vi "Get TimerDRV Period.vi"(11 "TimerDRV in":refnum<class "TimerDRV.lvclass">) -> (2 "TimerDRV Period":i64, 3 "TimerDRV out":refnum<class "TimerDRV.lvclass">)   [LabVIEW 2019, in "TimingDRV Engine.lvlib" / "TimerDRV.lvclass"]
uses:
  TimerDRV.lvclass
  TimerDRV.lvclass/TimerDRV.ctl
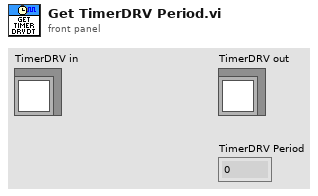
[diagram p1: front panel]
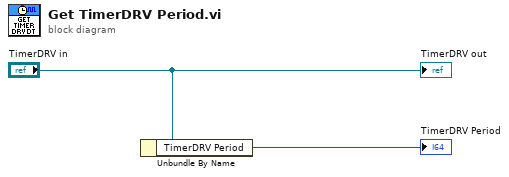
[diagram p0: block diagram]
diagram:
  n1 = Unbundle By Name("TimerDRV in") -> ("TimerDRV Period"=→"TimerDRV Period":i64)
  "TimerDRV out" <- "TimerDRV in"
